vi "timestamp_to_float.vi"() -> ()   [LabVIEW 2011]
panel:
  out "double precision float":dbl format="%#_13g"
  in  "Time Stamp":timestamp
  # "Not intended to be called, just an interactive calculator."
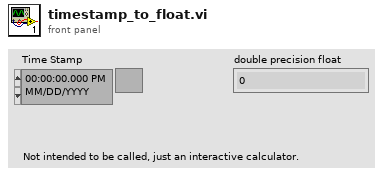
[diagram p1: front panel]
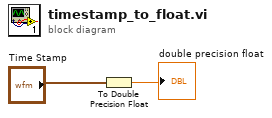
[diagram p0: block diagram]
diagram:
  n1 = To Double Precision Float(number="Time Stamp") -> (double precision float=→"double precision float":dbl)
